vi "Send Speed Message.vi"(6 "Data":u16 format="%x", 9 "Reset":bool) -> (2 "Bit 1 Out":bool, 3 "Bit 0 Out":bool)   [LabVIEW 2015]
uses:
  Protocol State.ctl
  <vilib>/rvi/Emulation/niFpgaSctlEmulationGetInTimedLoop.vi
  <vilib>/rvi/Emulation/niFpgaProcessEmulError.vi
panel:
  out "Timer":u32
  out "Temp Data":u16
  out "State":T1
  out "Bit Count":i32
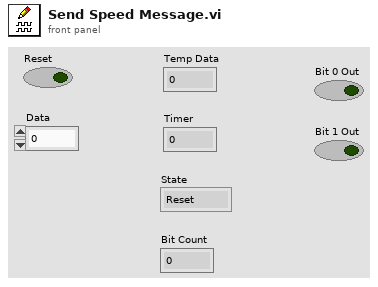
[diagram p1: front panel]
types:
  T1 = typedef "Protocol State.ctl" = enum16{"Reset", "Speed Pulse", "Delay After SP", "DP First Half", "Delay During First Half", "DP Second Half", "Delay During Second Half", "Idle"}
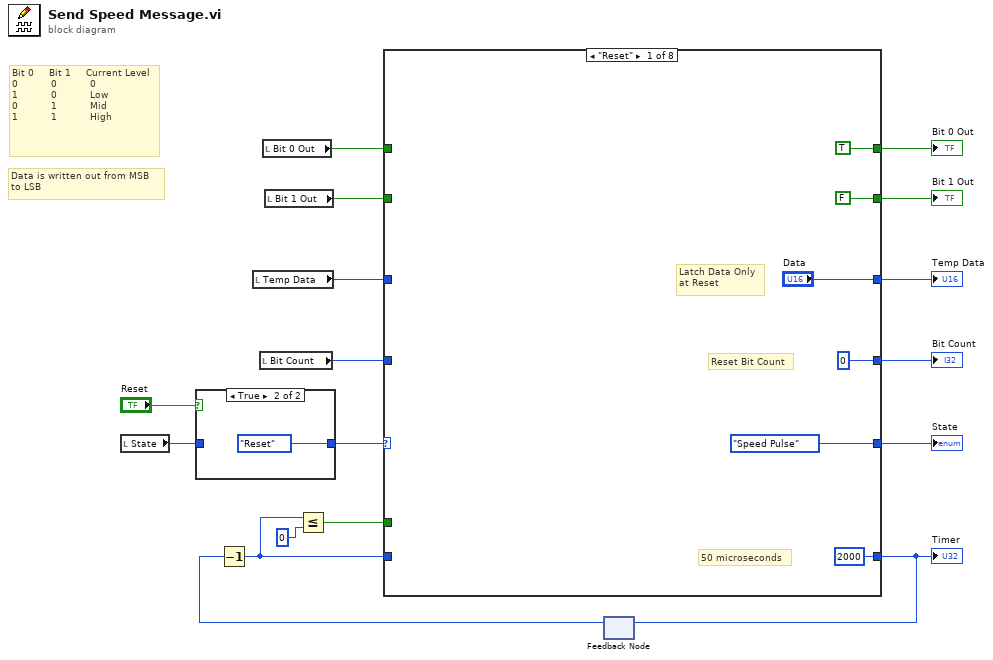
[diagram p0: block diagram]
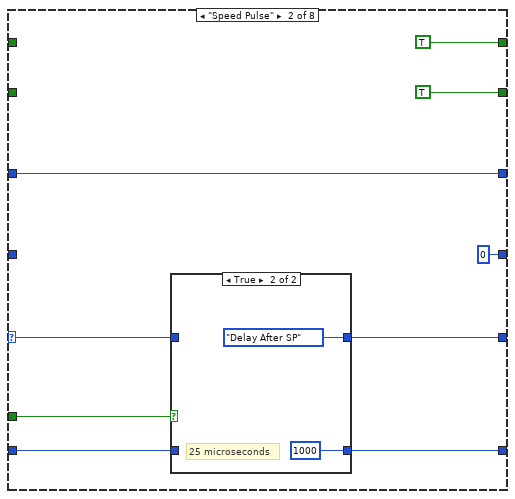
[diagram p3: hidden frame]
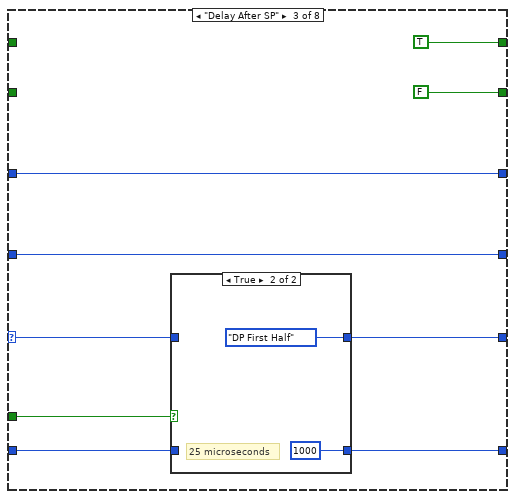
[diagram p5: hidden frame]
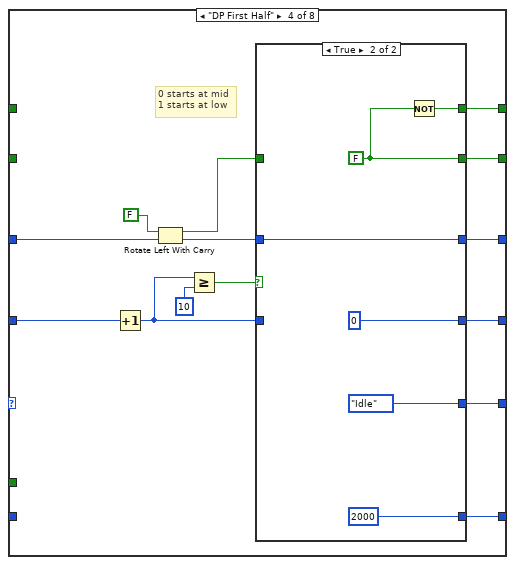
[diagram p7: hidden frame]
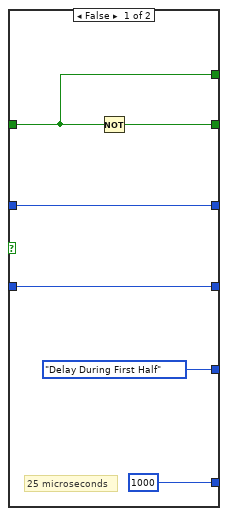
[diagram p8: hidden frame]
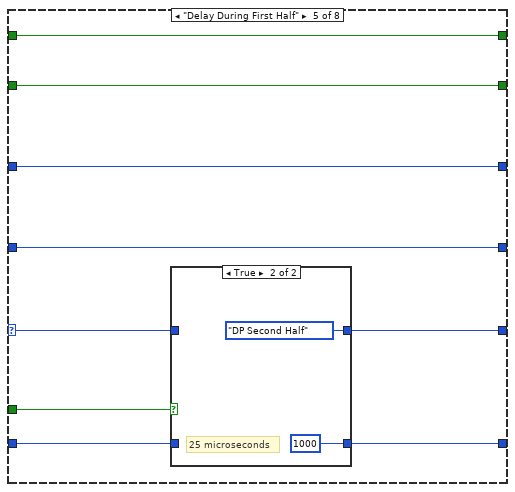
[diagram p9: hidden frame]
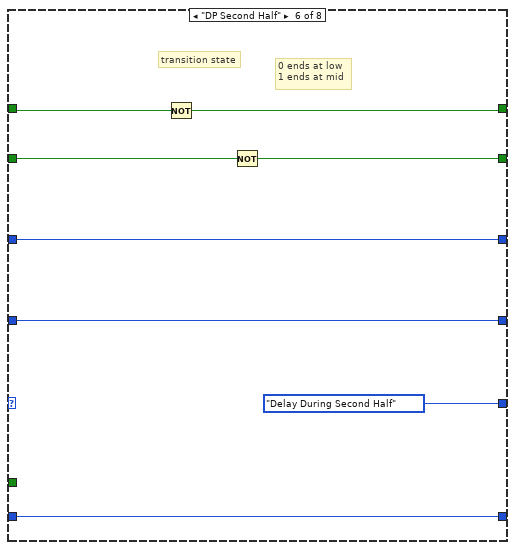
[diagram p11: hidden frame]
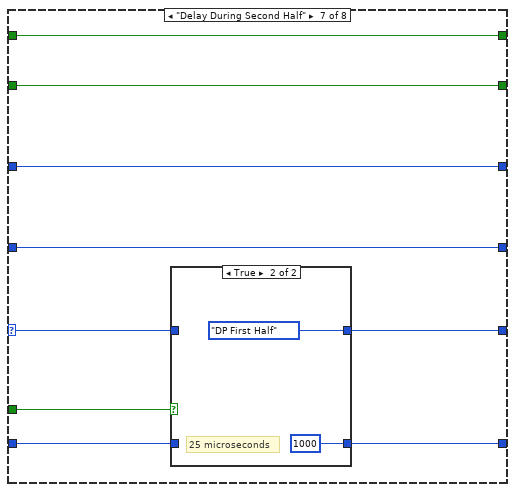
[diagram p12: hidden frame]
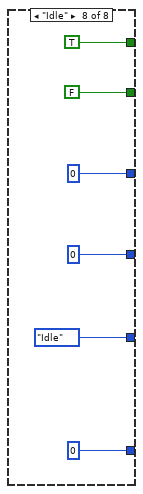
[diagram p14: hidden frame]
diagram:
  # "Data is written out from MSB\nto LSB"
  # "Bit 0     Bit 1     Current Level\n0           0           0\n1           0           Low\n0           1           Mid\n1           1           High"
  n1 = local read "State"() -> (w7:T1)
  n2 = case shown="True" "Reset" {
    tunnel: w7 -> [w18 _]
    tunnel: [w18 Protocol_State."Reset" ("State")] -> w12
    frame False {
    }
    frame True {
    }
  }
  n3 = local read "Temp Data"() -> (w5:u16)
  n4 = local read "Bit Count"() -> (w4:i32)
  n5 = local read "Bit 0 Out"() -> (w1:bool)
  n6 = local read "Bit 1 Out"() -> (w6:bool)
  n7 = feedback #1() -> (w9:u32)  [unwired: 1 in]
  n8 = Decrement(x=w9) -> (x-1=w3:u32)
  n9 = Less Or Equal?(x=w3, y=u32 0 ("x")) -> (x <= y?=w8:bool)
  n10 = case shown="\"Reset\"" w12 {
    selector: w12 -> [_ w29 w43 _ w83 _ w104 _]
    tunnel: [0 ("Bit Count") 0 ("Bit Count") w39 w64 w80 w95 w101 0 ("Bit Count")] -> w17
    tunnel: [FALSE ("carry") TRUE ("lsb carry out") FALSE ("msb carry out") w61 w79 w98 w99 FALSE ("Bit 0 Out")] -> w16
    tunnel: ["Data" w26 w40 w57 w81 w96 w102 u16 0 ("Data")] -> w15
    tunnel: [TRUE ("carry") TRUE ("carry") TRUE ("carry") w52 w78 w91 w100 TRUE ("carry")] -> w14
    tunnel: [Protocol_State."Speed Pulse" ("State") w28 w42 w56 w82 Protocol_State."Delay During Second Half" ("State") w103 Protocol_State."Idle" ("State")] -> w13
    tunnel: [u32 2000 ("Timer") w31 w45 w55 w85 w94 w106 u32 0 ("Timer")] -> w10
    tunnel: w3 -> [_ w30 w44 _ w84 w94 w105 _]
    tunnel: w8 -> [_ w32 w46 _ w86 _ w107 _]
    tunnel: w6 -> [_ _ _ _ w79 w93 w99 _]
    tunnel: w5 -> [_ w26 w40 w54 w81 w96 w102 _]
    tunnel: w4 -> [_ _ w39 w53 w80 w95 w101 _]
    tunnel: w1 -> [_ _ _ _ w78 w92 w100 _]
    frame "Reset" {
      # "Latch Data Only\nat Reset"
      # "50 microseconds"
      # "Reset Bit Count"
    }
    frame "Speed Pulse" {
      n11 = case shown="True" w32 {
        tunnel: [w36 u32 1000 ("Timer")] -> w31
        tunnel: w30 -> [w36 _]
        tunnel: w29 -> [w35 _]
        tunnel: [w35 Protocol_State."Delay After SP" ("State")] -> w28
        frame False {
        }
        frame True {
          # "25 microseconds"
        }
      }
    }
    frame "Delay After SP" {
      n12 = case shown="True" w46 {
        tunnel: [w49 u32 1000 ("Timer")] -> w45
        tunnel: w44 -> [w49 _]
        tunnel: w43 -> [w48 _]
        tunnel: [w48 Protocol_State."DP First Half" ("State")] -> w42
        frame False {
        }
        frame True {
          # "25 microseconds"
        }
      }
    }
    frame "DP First Half" {
      # "0 starts at mid \n1 starts at low"
      n13 = Increment(x=w53) -> (x+1=w58:i32)
      n14 = Rotate Left With Carry(2:w54, 3:FALSE ("carry")) -> (0:w59:u16, 1:w62:bool)
      n15 = Greater Or Equal?(x=w58, y=10 ("x")) -> (x >= y?=w65:bool)
      n16 = case shown="True" w65 {
        tunnel: [w71 0] -> w64
        tunnel: w58 -> [w71 _]
        tunnel: [w67 w73] -> w61
        tunnel: w62 -> [w66 _]
        tunnel: w59 -> [w70 w76]
        tunnel: [w70 w76] -> w57
        tunnel: [Protocol_State."Delay During First Half" ("State") Protocol_State."Idle" ("State")] -> w56
        tunnel: [u32 1000 ("Timer") u32 2000 ("Timer")] -> w55
        tunnel: [w66 w72] -> w52
        frame False {
          # "25 microseconds"
          n17 = Not(x=w66) -> (.not. x?=w67:bool)
        }
        frame True {
          w73 = FALSE ("msb carry out")
          n18 = Not(x=w73) -> (.not. x?=w72:bool)
        }
      }
    }
    frame "Delay During First Half" {
      n19 = case shown="True" w86 {
        tunnel: [w88 u32 1000 ("Timer")] -> w85
        tunnel: w84 -> [w88 _]
        tunnel: w83 -> [w87 _]
        tunnel: [w87 Protocol_State."DP Second Half" ("State")] -> w82
        frame False {
        }
        frame True {
          # "25 microseconds"
        }
      }
    }
    frame "DP Second Half" {
      # "0 ends at low \n1 ends at mid"
      # "transition state"
      n20 = Not(x=w92) -> (.not. x?=w91:bool)
      n21 = Not(x=w93) -> (.not. x?=w98:bool)
    }
    frame "Delay During Second Half" {
      n22 = case shown="True" w107 {
        tunnel: [w109 u32 1000 ("Timer")] -> w106
        tunnel: w105 -> [w109 _]
        tunnel: w104 -> [w108 _]
        tunnel: [w108 Protocol_State."DP First Half" ("State")] -> w103
        frame False {
        }
        frame True {
          # "25 microseconds"
        }
      }
    }
    frame "Idle" {
    }
  }
  "Bit Count" <- w17
  "Bit 1 Out" <- w16
  "State" <- w13
  "Temp Data" <- w15
  "Timer" <- w10
  "Bit 0 Out" <- w14
  n23 = feedback-in #1(w10) -> ()
